vi "Remove Placeholder.vi"(8 "error in (no error)":errorcluster, 11 "Entity Class":refnum<vi>) -> (0 "error out":errorcluster)   [LabVIEW 2020, in "Conditum-Tools.lvlib" / "Entity Editor.lvclass"]
uses:
  Entity Editor.lvclass
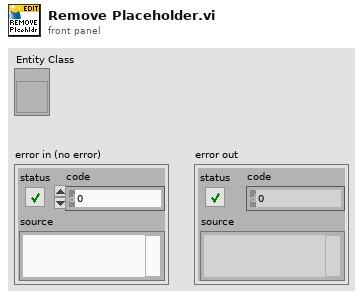
[diagram p1: front panel]
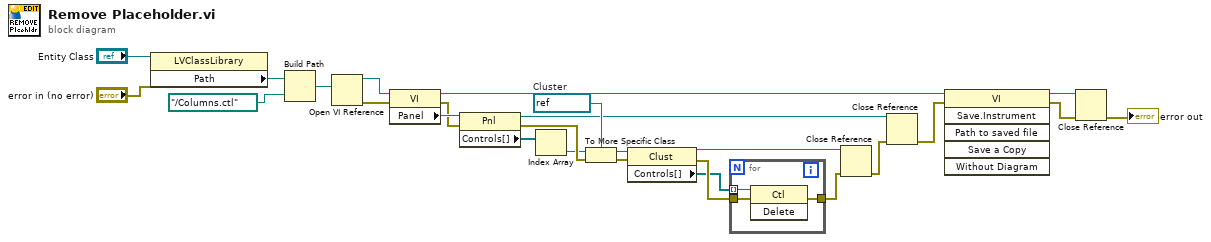
[diagram p0: block diagram]
diagram:
  w17 = refnum<vi> refnum  # Cluster
  n1 = property class="LVClassLibrary"(reference="Entity Class", error in="error in (no error)") -> ("Path"=w25:path)  [unwired: 2 out]
  n2 = Build Path(base path=w25, name or relative path=path "../Columns.ctl") -> (appended path=w23:path)
  n3 = Open VI Reference(vi path=w23) -> (vi reference=w12:refnum<vi>, error out=w11:errorcluster)  [unwired: 5 in]
  n4 = property class="VI"(reference=w12, error in=w11) -> (reference out=w4:refnum<vi>, error out=w14:errorcluster, "Panel"=w20:refnum<vi>)
  n5 = property class="Pnl"(reference=w20, error in=w14) -> (reference out=w8:refnum<vi>, error out=w22:errorcluster, "Controls[]"=w19:refnum<vi>[])
  n6 = Index Array(array=w19) -> (element=w18:refnum<vi>)  [unwired: 1 in]
  n7 = To More Specific Class(target class=w17, reference=w18, error in=w22) -> (specific class reference=w16:refnum<vi>, error out=w13:errorcluster)
  n8 = property class="Clust"(reference=w16, error in=w13) -> (reference out=w9:refnum<vi>, error out=w21:errorcluster, "Controls[]"=w15:refnum<vi>[])
  n9 = for {
    tunnel: w15 -> [w29] mode=indexing
    tunnel: [w28] -> w10
    tunnel: w21 -> [w27]
    n10 = invoke class="Ctl" method="Delete"(reference=w29, error in=w27) -> (error out=w28:errorcluster)  [unwired: 1 in, 2 out]
  }
  n11 = Close Reference(reference=w9, error in (no error)=w10) -> (error out=w7:errorcluster)
  n12 = Close Reference(reference=w8, error in (no error)=w7) -> (error out=w3:errorcluster)
  n13 = invoke class="VI" method="Save.Instrument"(reference=w4, error in=w3) -> (reference out=w2:refnum<vi>, error out=w1:errorcluster)  [unwired: 4 in, 4 out]
  n14 = Close Reference(reference=w2, error in (no error)=w1) -> (error out=→"error out":errorcluster)
